vi "ZZ.vi"(1 "P":cdb[](array[numeric])) -> (0 "PP*":dbl[](array[numeric]))   [LabVIEW 2014]
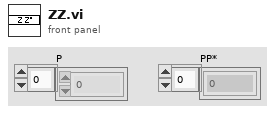
[diagram p1: front panel]
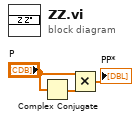
[diagram p0: block diagram]
diagram:
  n1 = Complex Conjugate(1:"P") -> (0:w1:cdb[])
  n2 = Multiply(x="P", y=w1) -> (x*y=→"PP*":cdb[])
